vi "VsEP-Analyze.vi"(0 "Neural (uV)":dbl[](array[numeric]), 2 "Runtime":T1, 5 "microphonic (uV)":dbl[](array[numeric]), 7 "Averaging data":cluster{i32, i32}, 9 "Normalize individual?":bool, 11 "error in":errorcluster, 12 "Analysis":T3, 13 "Graphs":T2) -> (14 "Analysis out":T3, 15 "error out":errorcluster)   [LabVIEW 2020]
uses:
  Typedefs/VsEP-Analysis State.ctl
  Typedefs/VsEP-Graph Controls.ctl
  Typedefs/VsEP-Runtime Data.ctl
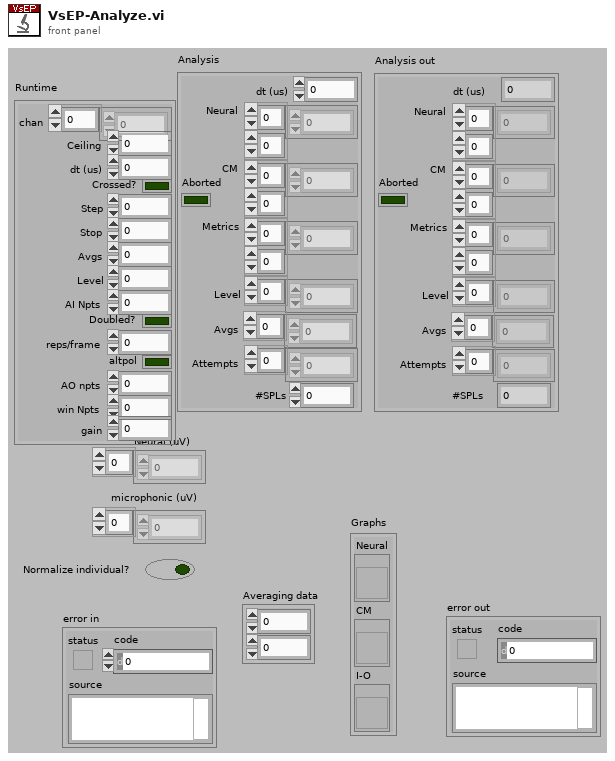
[diagram p1: front panel]
types:
  T1 = typedef "VsEP-Runtime Data.ctl" = cluster{"chan":i32[], "Ceiling":dbl, "dt (us)":dbl, "Crossed?":bool, "Step":dbl, "Stop":i32, "Avgs":i32, "Level":dbl, "AI Npts":i32, "Doubled?":bool, "reps/frame":i32, "altpol":bool, "AO npts":i32, "win Npts":i32, "gain":dbl}
  T2 = typedef "VsEP-Graph Controls.ctl" = cluster{"Neural":refnum<vi>, "CM":refnum<vi>, "I-O":refnum<vi>}
  T3 = typedef "VsEP-Analysis State.ctl" = cluster{"dt (us)":dbl, "Neural":dbl[][], "CM":dbl[][], "Metrics":dbl[][], "Level":dbl[], "Avgs":i32[], "Attempts":i32[], "Aborted":bool, "#SPLs":i32}
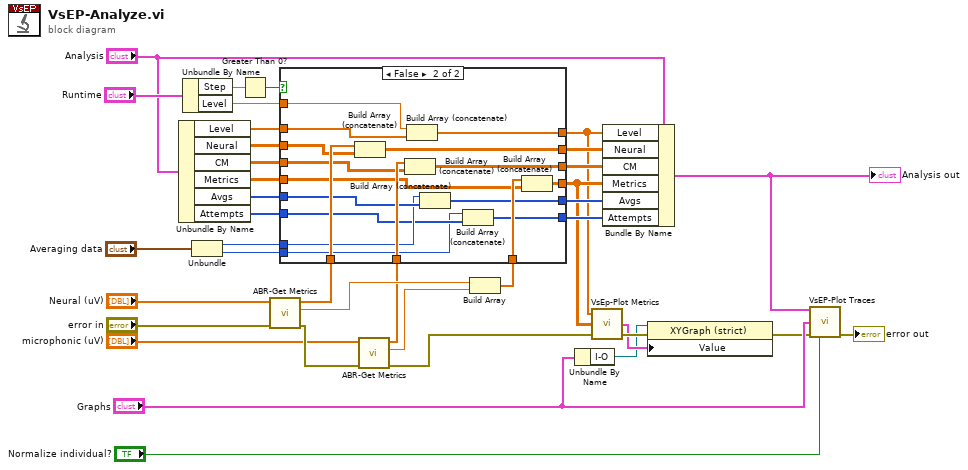
[diagram p0: block diagram]
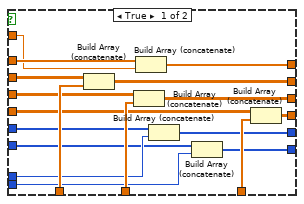
[diagram p2: hidden frame]
diagram:
  n1 = Unbundle By Name("Analysis") -> ("Level"=w27:dbl[], "Neural"=w32:dbl[][], "CM"=w31:dbl[][], "Metrics"=w30:dbl[][], "Avgs"=w25:i32[], "Attempts"=w21:i32[])
  n2 = Unbundle By Name("Runtime") -> ("Step"=w15:dbl, "Level"=w26:dbl)
  n3 = Unbundle("Averaging data") -> (w23:i32, w19:i32)
  n4 = Greater Than 0?(x=w15) -> (x > 0?=w14:bool)
  n5 = call "ABR-Get Metrics.vi"("error in (no error)"="error in", "Data in"="Neural (uV)") -> ("error out"=w29:errorcluster, "spread value"=w38:dbl, "Data out"=w36:dbl[])  [unwired: 7 in]
  n6 = call "ABR-Get Metrics.vi"("error in (no error)"=w29, "Data in"="microphonic (uV)") -> ("error out"=w2:errorcluster, "spread value"=w34:dbl, "Data out"=w35:dbl[])  [unwired: 7 in]
  n7 = Build Array(w38, w34) -> (w37:dbl[])
  n8 = case shown="False" w14 {
    tunnel: w37 -> [w56 w74]
    tunnel: w36 -> [w55 w73]
    tunnel: w35 -> [w54 w72]
    tunnel: w32 -> [w53 w71]
    tunnel: w31 -> [w52 w70]
    tunnel: w30 -> [w51 w69]
    tunnel: [w50 w68] -> w13
    tunnel: [w49 w67] -> w12
    tunnel: [w48 w66] -> w11
    tunnel: w27 -> [w47 w65]
    tunnel: [w46 w64] -> w1
    tunnel: w26 -> [w45 w63]
    tunnel: w25 -> [w44 w62]
    tunnel: w23 -> [w43 w61]
    tunnel: [w42 w60] -> w22
    tunnel: w21 -> [w41 w59]
    tunnel: [w40 w58] -> w20
    tunnel: w19 -> [w39 w57]
    frame True {
      n9 = Build Array (concatenate)(w53, w55) -> (w50:dbl[][])
      n10 = Build Array (concatenate)(w52, w54) -> (w49:dbl[][])
      n11 = Build Array (concatenate)(w47, w45) -> (w46:dbl[])
      n12 = Build Array (concatenate)(w44, w43) -> (w42:i32[])
      n13 = Build Array (concatenate)(w41, w39) -> (w40:i32[])
      n14 = Build Array (concatenate)(w51, w56) -> (w48:dbl[][])
    }
    frame False {
      n15 = Build Array (concatenate)(w73, w71) -> (w68:dbl[][])
      n16 = Build Array (concatenate)(w72, w70) -> (w67:dbl[][])
      n17 = Build Array (concatenate)(w63, w65) -> (w64:dbl[])
      n18 = Build Array (concatenate)(w61, w62) -> (w60:i32[])
      n19 = Build Array (concatenate)(w57, w59) -> (w58:i32[])
      n20 = Build Array (concatenate)(w74, w69) -> (w66:dbl[][])
    }
  }
  n21 = Unbundle By Name("Graphs") -> ("I-O"=w8:refnum<vi>)
  n22 = call "VsEp-Plot Metrics.vi"("error in (no error)"=w2, "metrics"=w11, "level"=w1) -> ("error out"=w10:errorcluster, "appended array"=w9:cluster{"array":ext[], "array":ext[]}[])  [unwired: 1 in]
  n23 = Bundle By Name(cluster="Analysis", "Level"=w1, "Neural"=w13, "CM"=w12, "Metrics"=w11, "Avgs"=w22, "Attempts"=w20) -> (w7:T3)
  "Analysis out" <- w7
  n24 = property class="XYGraph (strict)"(reference=w8, error in=w10, "Value"=w9) -> (error out=w5:errorcluster)  [unwired: 1 out]
  n25 = call "VsEP-Plot Traces.vi"("Analysis"=w7, "Graphs"="Graphs", "error in"=w5, "Normalize individual?"="Normalize individual?") -> ("error out"=→"error out":errorcluster)  [unwired: 11 in]
